vi "Append to Stdout.vi"   [LabVIEW 2015, in "StdOut Operations.lvlib"]
uses:
  StdOut Operations.lvlib
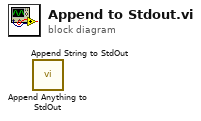
[diagram p0: block diagram]
diagram:
  n1 = call "Append Anything to StdOut.vi"() -> ()  [unwired: 7 in, 1 out]
  n2 = call "Append String to StdOut.vi"() -> ()  [unwired: 7 in, 1 out]
